vi "Index By WB.vi"(1 "Wet Bulb Temp [DegF]":dbl) -> (0 "WB Index":dbl)   [LabVIEW 2020]
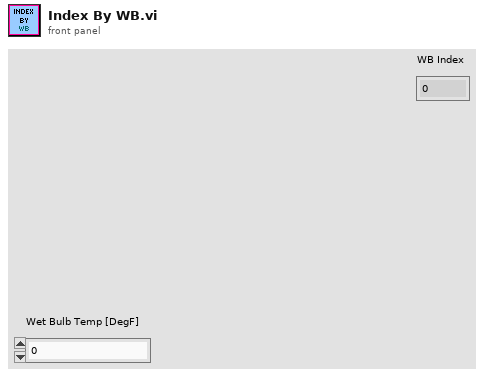
[diagram p1: front panel]
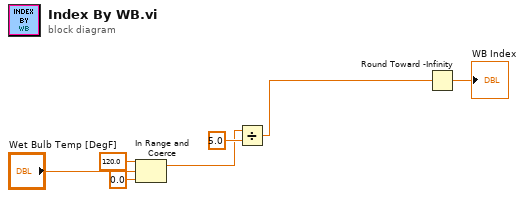
[diagram p0: block diagram]
diagram:
  n1 = In Range and Coerce(upper limit=120.0, x="Wet Bulb Temp [DegF]", lower limit=0.0) -> (coerced(x)=w4:dbl)  [unwired: 1 out]
  n2 = Divide(x=w4, y=5.0) -> (x/y=w1:dbl)
  n3 = Round Toward -Infinity(1:w1) -> (0:→"WB Index":dbl)
